vi "VI_botões_Dashboard.vi"(10 "Switch_Scale":T1, 11 "NavX_Reset":bool) -> ()   [LabVIEW 2017]
uses:
  <vilib>/Rock Robotics/Network Tables/NT Write Boolean.vi
  <vilib>/Rock Robotics/Network Tables/NT Write Number.vi
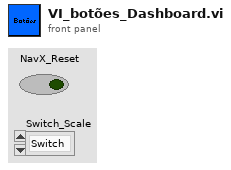
[diagram p1: front panel]
types:
  T1 = typedef "Control 2.ctl" = enum16{"Switch", "Scale"}
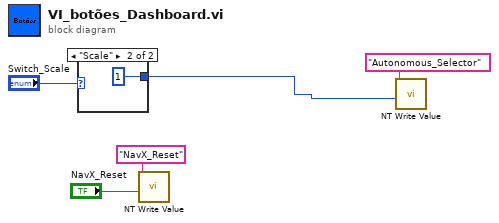
[diagram p0: block diagram]
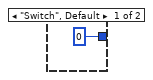
[diagram p2: hidden frame]
diagram:
  n1 = case shown="\"Scale\"" "Switch_Scale" {
    tunnel: [0 1] -> w1
    frame "Switch", Default {
    }
    frame "Scale" {
    }
  }
  n2 = call-poly <vilib>:"NT Write Value.vi"("Boolean"="NavX_Reset", "Name"="NavX_Reset") -> ()  [unwired: 9 in, 1 out]
  n3 = call-poly <vilib>:"NT Write Value.vi"("Numeric"=w1, "Name"="Autonomous_Selector") -> ()  [unwired: 9 in, 1 out]
